vi "GTSINDICATOR.vi"(11 "Numeric":u8) -> (0 "Boolean array[3]":bool, 1 "Boolean array[2]":bool, 2 "Boolean array[1]":bool, 3 "Boolean array[0]":bool, 4 "Boolean array[5]":bool, 5 "Boolean array[4]":bool, 6 "Boolean array[7]":bool, 7 "Boolean array[6]":bool)   [LabVIEW 2011]
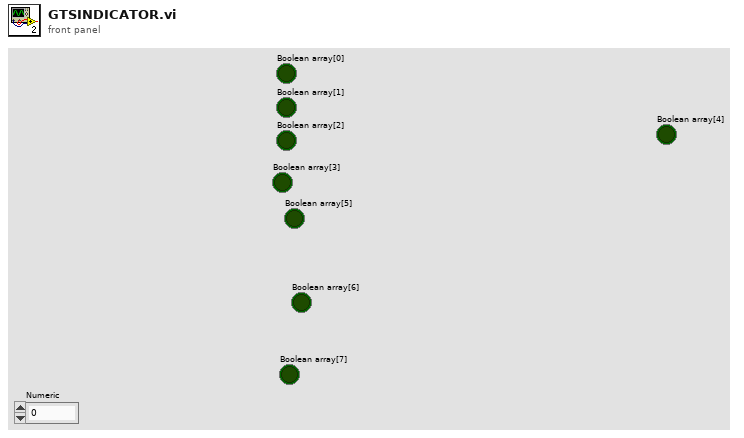
[diagram p1: front panel]
types:
  T1 = cluster{"Boolean array[0]":bool, "Boolean array[1]":bool, "Boolean array[2]":bool, "Boolean array[3]":bool, "Boolean array[4]":bool, "Boolean array[5]":bool, "Boolean array[6]":bool, "Boolean array[7]":bool, "Boolean array[8]":bool}
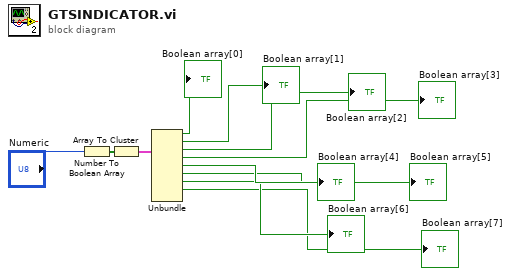
[diagram p0: block diagram]
diagram:
  n1 = Number To Boolean Array(number="Numeric") -> (Boolean array=w10:bool[])
  n2 = Array To Cluster(array=w10) -> (cluster=w9:T1)
  n3 = Unbundle(w9) -> ("Boolean array[0]"=→"Boolean array[0]":bool, "Boolean array[1]"=→"Boolean array[1]":bool, "Boolean array[2]"=→"Boolean array[2]":bool, "Boolean array[3]"=→"Boolean array[3]":bool, "Boolean array[4]"=→"Boolean array[4]":bool, "Boolean array[5]"=→"Boolean array[5]":bool, "Boolean array[6]"=→"Boolean array[6]":bool, "Boolean array[7]"=→"Boolean array[7]":bool)  [unwired: 1 out]
